vi "Periodic Tasks.vi"(8 "error in":errorcluster) -> ()   [LabVIEW 2015]
doc: "This VI runs in parallel to other tasks. It can contain as many user-defined periodic loops as you need. These can carry out PID or other sorts of timed response."
uses:
  <vilib>/Rock Robotics/WPI/Solenoid/WPI_SolenoidValue.ctl
  Robot Global Data.vi
  <vilib>/Rock Robotics/Network Tables/NT Write Boolean.vi
  <vilib>/Rock Robotics/Network Tables/NT Write Number.vi
  <vilib>/Rock Robotics/WPI/Solenoid/WPI_SolenoidSetEnum.vi
  <vilib>/Rock Robotics/Network Tables/NT Write Raw.vi
  <vilib>/Rock Robotics/Network Tables/NT Write Numeric Array.vi
  <vilib>/Rock Robotics/Network Tables/NT Read Boolean.vi
  <vilib>/Rock Robotics/WPI/Utilities/WPI_GetSetVariantRefNum.vi
panel:
  in  "Trim Speed":dbl
  in  "Rate":dbl min=0.0 max=0.1 step=0.001
  out "Ramp Up":dbl(knob) scale=0.0..1.0
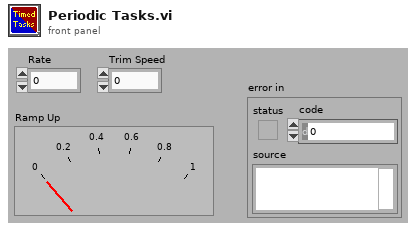
[diagram p1: front panel]
types:
  T1 = typedef "WPI_SolenoidValue.ctl" = enum16{"Off", "On", "Forward", "Reverse"}
  T2 = typedef "WPI_SolenoidDevRef.ctl" = cluster{"DevStatus":errorcluster, "Pneumatics Control Module":u8, "Forward Solenoid Channel":T3, "Reverse Solenoid Channel":T3}
  T3 = typedef "WPI_SolenoidChannel.ctl" = enum8{"Solenoid 0", "Solenoid 1", "Solenoid 2", "Solenoid 3", "Solenoid 4", "Solenoid 5", "Solenoid 6", "Solenoid 7", "Invalid"}
  T4 = typedef "WPI_DigitalInputDevRef.ctl" = cluster{"DevStatus":errorcluster, "DIO Channel":T5}
  T5 = typedef "FPGA_DIOChannel.ctl" = enum8{"DIO 0", "DIO 1", "DIO 2", "DIO 3", "DIO 4", "DIO 5", "DIO 6", "DIO 7", "DIO 8", "DIO 9", "DIO MXP 0", "DIO MXP 1", "DIO MXP 2", "DIO MXP 3", "DIO MXP 4", "DIO MXP 5", "DIO MXP 6", "DIO MXP 7", "DIO MXP 8", "DIO MXP 9", "DIO MXP 10", "DIO MXP 11", "DIO MXP 12", "DIO MXP 13", "DIO MXP 14", "DIO MXP 15", "Invalid"}
  T6 = typedef "WPI_MotorControlDeviceRef.ctl" = cluster{"DeviceStatus":errorcluster, "Type":T7, "PWM":cluster{"PWM Channel":T8, "DeadBand":T9}, "CAN":cluster{"Device Number":u8, "Control Mode":T10, "Semaphore":T11, "Max Vout":dbl, "TalonSRX Control Mode":T12}, "Invert":bool}
  T7 = typedef "WPI_MotorControlType.ctl" = enum16{"PWM", "CAN", "CANTalonSRX"}
  T8 = typedef "FPGA_DIOPWMChannel.ctl" = enum8{"PWM 0", "PWM 1", "PWM 2", "PWM 3", "PWM 4", "PWM 5", "PWM 6", "PWM 7", "PWM 8", "PWM 9", "PWM MXP 0", "PWM MXP 1", "PWM MXP 2", "PWM MXP 3", "PWM MXP 4", "PWM MXP 5", "PWM MXP 6", "PWM MXP 7", "PWM MXP 8", "PWM MXP 9", "Invalid"}
  T9 = typedef "WPI_PWMDeadband.ctl" = cluster{"Name":string, "maxPositivePwm":i32, "minPositivePwm":i32, "centerPwm":i32, "maxNegativePwm":i32, "minNegativePwm":i32, "angularRange":u16}
  T10 = typedef "WPI_CANJaguar_ControlMode.ctl" = enum8{"Percent VBus", "Current", "Speed", "Position", "Voltage"}
  T11 = typedef "Semaphore RefNum" = refnum<k1>
  T12 = typedef "WPI_CANTalonSRX_APIControlMode.ctl" = enum8{"Percent VBus", "Speed", "Position", "Slave", "Unchanged / Invalid", "Voltage Compensation", "Current", "Motion Profile"}
  T13 = typedef "WPI_RobotDriveDevRef.ctl" = cluster{"DevStatus":errorcluster, "Motors[]":T6[], "Square Inputs":bool, "Max Output":dbl}
  T14 = typedef "WPI_DriverStationRobotMode2.ctl" = enum16{"Autonomous Disabled", "Autonomous Enabled", "Teleop Disabled", "Teleop Enabled", "Disconnected", "Finish", "Test Disabled", "Test Enabled", "Emergency Stopped"}
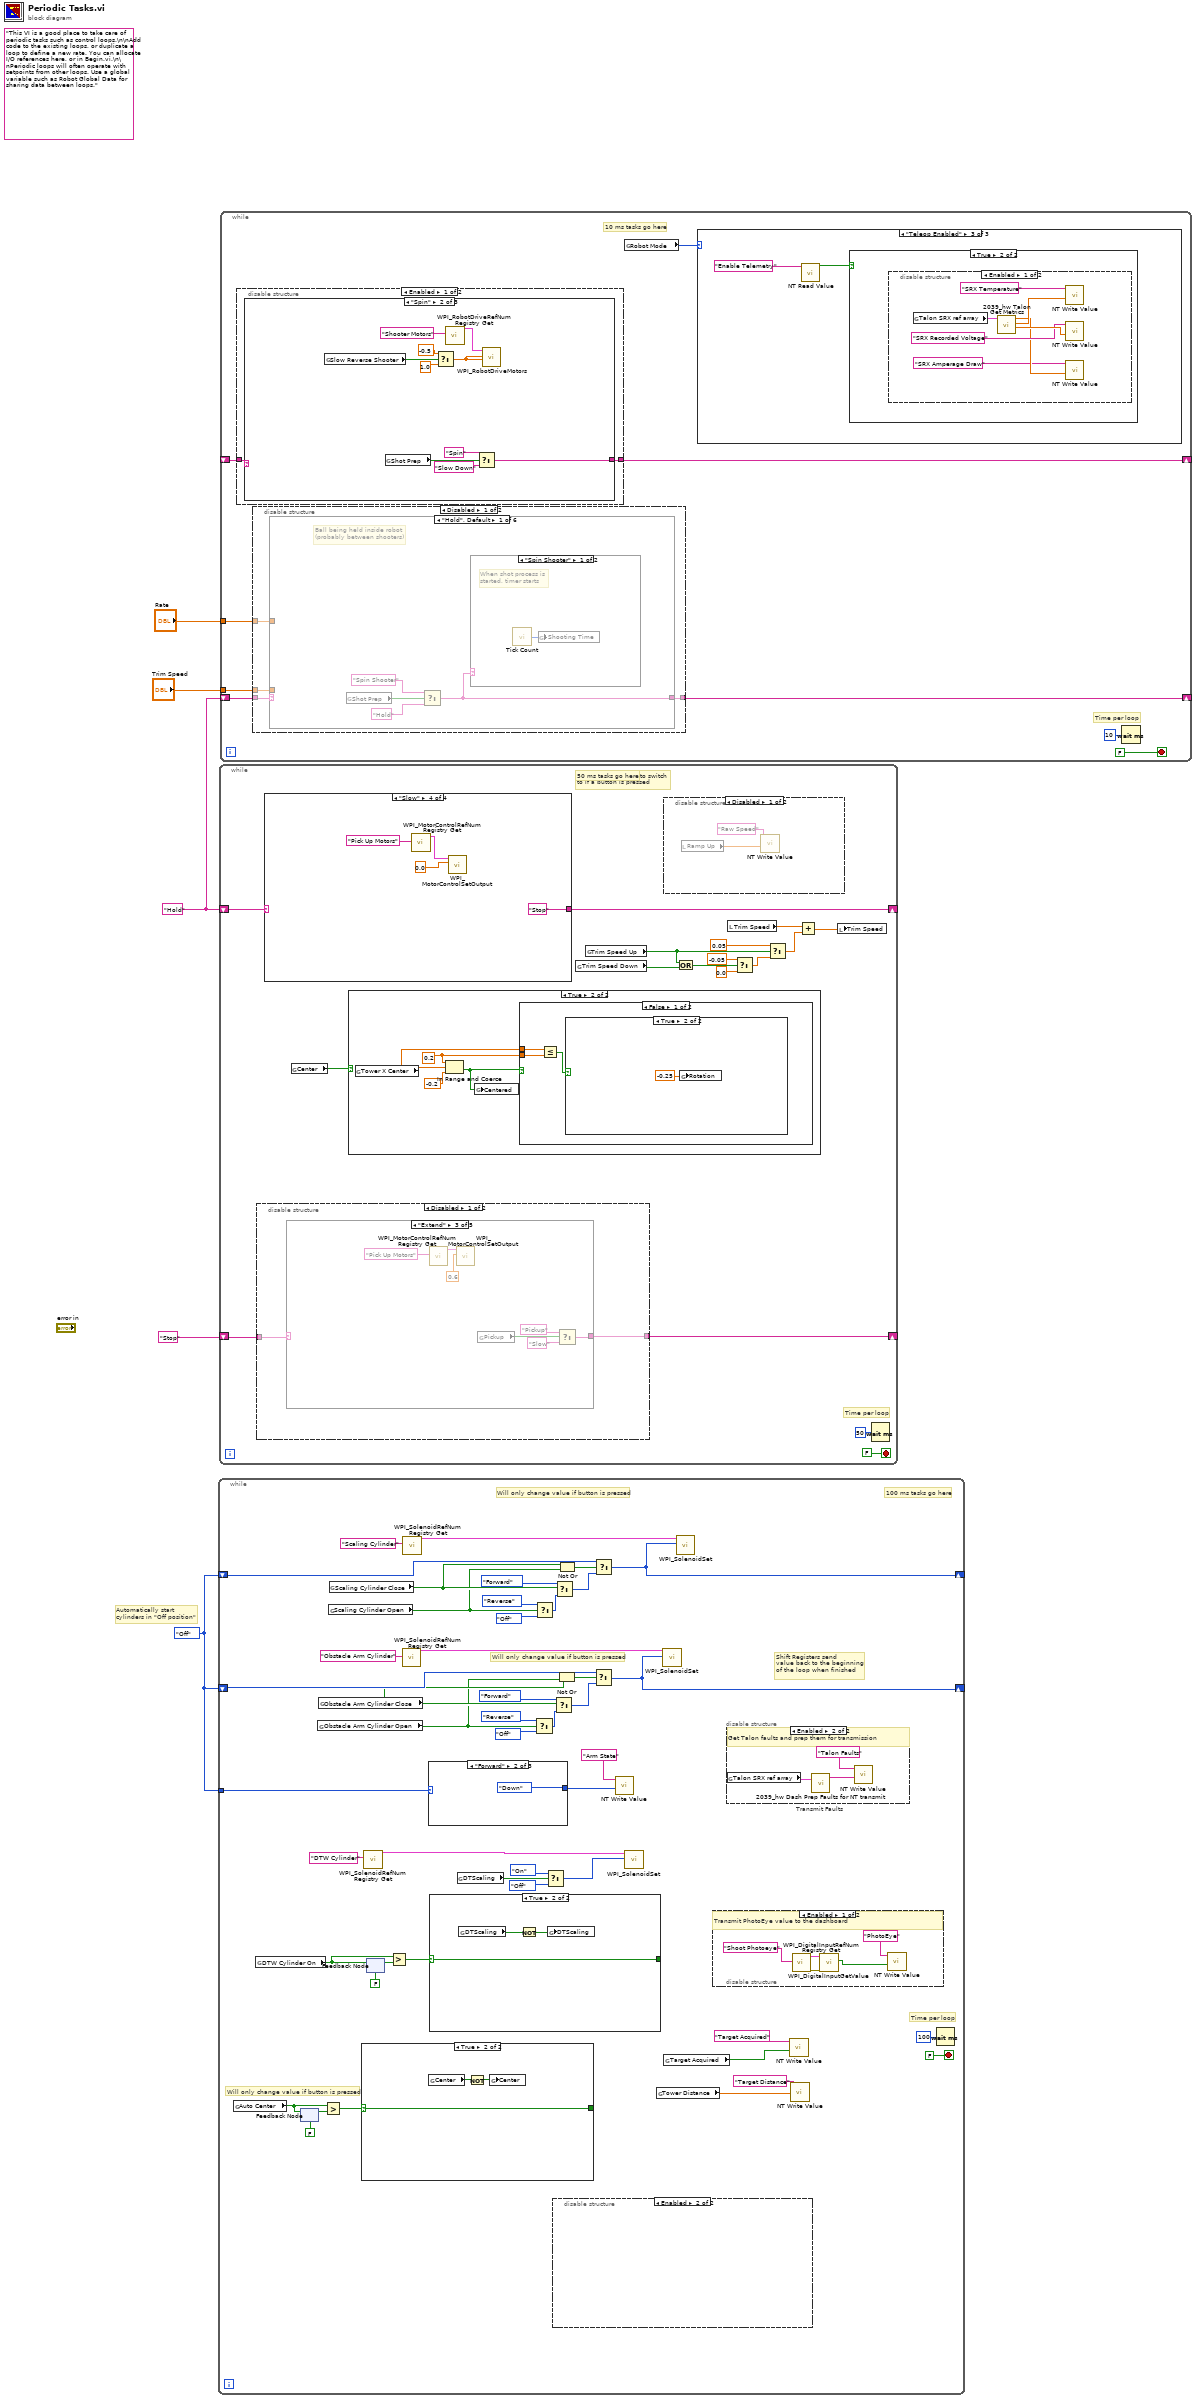
[diagram p0: block diagram]
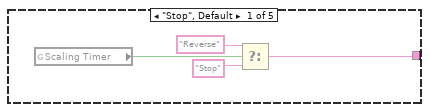
[diagram p2: hidden frame]
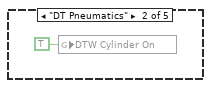
[diagram p3: hidden frame]
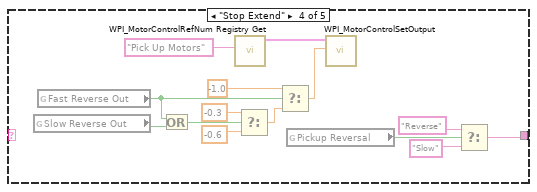
[diagram p4: hidden frame]
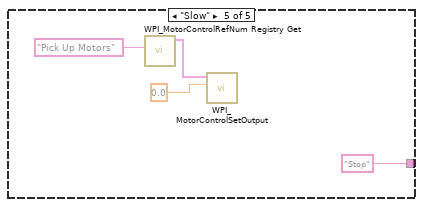
[diagram p5: hidden frame]
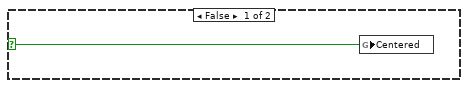
[diagram p8: hidden frame]
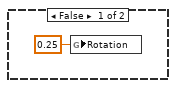
[diagram p9: hidden frame]
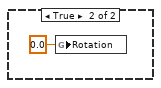
[diagram p10: hidden frame]
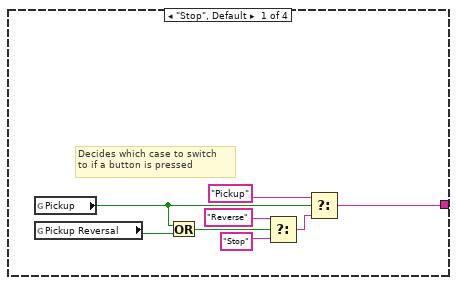
[diagram p11: hidden frame]
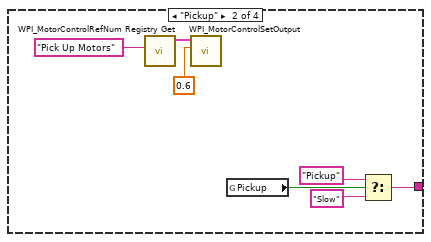
[diagram p12: hidden frame]
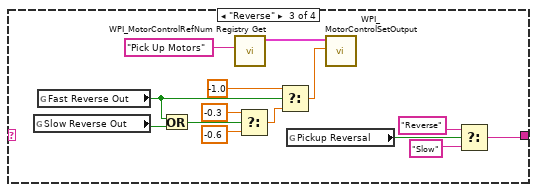
[diagram p13: hidden frame]
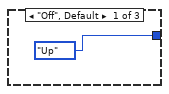
[diagram p18: hidden frame]
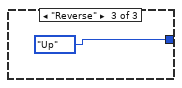
[diagram p19: hidden frame]
diagram:
  w2 = WPI_SolenoidValue."Off" ("Value")
  w4 = "Hold"
  (unwired) "This VI is a good place to take care of periodic tasks such as control loops.\n\nAdd code to the existing loops, or duplicate a loop to define a new rate. You can allocate I/O references here, or in Begin.vi.\n\nPeriodic loops will often operate with setpoints from other loops. Use a global variable such as Robot Global Data for sharing data between loops."
  # "Automatically start \ncylinders in \"Off position\""
  n1 = while {
    shift-right: [w50] -> _
    shift-left: w2 -> [w49]
    shift-right: [w44] -> _
    shift-left: w2 -> [w43]
    tunnel: w2 -> [w23]
    stop <- FALSE stop-if-true
    # "Will only change value if button is pressed"
    # "Will only change value if button is pressed"
    # "Will only change value if button is pressed"
    # "Shift Registers send\nvalue back to the beginning\nof the loop when finished"
    # "Time per loop"
    # "100 ms tasks go here"
    n2 = global read "Robot Global Data.vi" "Auto Center"() -> (w18:bool)
    n3 = global read "Robot Global Data.vi" "DTW Cylinder On"() -> (w9:bool)
    n4 = feedback-in #1(w18) -> ()
    n5 = feedback #1(FALSE ("Auto Center")) -> (w19:bool)
    n6 = global read "Robot Global Data.vi" "Obstacle Arm Cylinder Open"() -> (w33:bool)
    n7 = global read "Robot Global Data.vi" "Obstacle Arm Cylinder Close"() -> (w34:bool)
    n8 = Greater?(x=w18, y=w19) -> (0:w20:bool)
    n9 = global read "Robot Global Data.vi" "Scaling Cylinder Open"() -> (w12:bool)
    n10 = global read "Robot Global Data.vi" "Scaling Cylinder Close"() -> (w24:bool)
    n11 = case shown="True" w20 {
      selector: w20 -> [w68 w71]
      tunnel: [w68 w71] -> _
      frame False {
      }
      frame True {
        n12 = global read "Robot Global Data.vi" "Center"() -> (w69:bool)
        n13 = Not(x=w69) -> (.not. x?=w70:bool)
        n14 = global write "Robot Global Data.vi" "Center"(w70) -> ()
      }
    }
    n15 = call <vilib>:"WPI_SolenoidRefNum Registry Get.vi"("refnum name"="DTW Cylinder") -> ("SolenoidDevRef"=w47:T2)  [unwired: 9 in, 1 out]
    n16 = feedback #2(FALSE ("Auto Center")) -> (w11:bool)
    n17 = feedback-in #2(w9) -> ()
    n18 = Greater?(x=w9, y=w11) -> (0:w6:bool)
    n19 = call <vilib>:"WPI_SolenoidRefNum Registry Get.vi"("refnum name"="Obstacle Arm Cylinder") -> ("SolenoidDevRef"=w37:T2)  [unwired: 9 in, 1 out]
    n20 = call <vilib>:"WPI_SolenoidRefNum Registry Get.vi"("refnum name"="Scaling Cylinder") -> ("SolenoidDevRef"=w27:T2)  [unwired: 9 in, 1 out]
    n21 = case shown="\"Forward\"" w23 {
      tunnel: [enum16{"Up", "Down"}."Up" enum16{"Up", "Down"}."Down" enum16{"Up", "Down"}."Up"] -> w22
      frame "Off", Default {
      }
      frame "Forward" {
      }
      frame "Reverse" {
      }
    }
    n22 = case shown="True" w6 {
      selector: w6 -> [w53 w56]
      tunnel: [w53 w56] -> _
      frame False {
      }
      frame True {
        n23 = global read "Robot Global Data.vi" "DTScaling"() -> (w54:bool)
        n24 = Not(x=w54) -> (.not. x?=w55:bool)
        n25 = global write "Robot Global Data.vi" "DTScaling"(w55) -> ()
      }
    }
    n26 = global read "Robot Global Data.vi" "DTScaling"() -> (w7:bool)
    n27 = Select(t=WPI_SolenoidValue."Reverse" ("Value"), s=w33, f=WPI_SolenoidValue."Off" ("Value")) -> (s? t:f=w39:T1)
    n28 = Select(t=WPI_SolenoidValue."Reverse" ("Value"), s=w12, f=WPI_SolenoidValue."Off" ("Value")) -> (s? t:f=w29:T1)
    n29 = Select(t=WPI_SolenoidValue."On" ("Value"), s=w7, f=WPI_SolenoidValue."Off" ("Value")) -> (s? t:f=w8:T1)
    n30 = disable-structure shown="Enabled" {
      frame Disabled {
      }
      frame Enabled {
      }
    }
    n31 = Select(t=WPI_SolenoidValue."Forward" ("Value"), s=w34, f=w39) -> (s? t:f=w36:T1)
    n32 = Select(t=WPI_SolenoidValue."Forward" ("Value"), s=w24, f=w29) -> (s? t:f=w26:T1)
    n33 = Not Or(1:w33, 2:w34) -> (0:w35:bool)
    n34 = Not Or(1:w12, 2:w24) -> (0:w25:bool)
    n35 = Select(t=w43, s=w35, f=w36) -> (s? t:f=w44:T1)
    n36 = Select(t=w49, s=w25, f=w26) -> (s? t:f=w50:T1)
    n37 = call-poly <vilib>:"NT Write Value.vi"("Numeric"=w22, "Name"="Arm State") -> ()  [unwired: 9 in, 1 out]
    n38 = call-poly <vilib>:"WPI_SolenoidSet.vi"("Value"=w8, "SolenoidDevRef"=w47) -> ()  [unwired: 1 in, 9 out]
    n39 = global read "Robot Global Data.vi" "Tower Distance"() -> (w14:dbl)
    n40 = call-poly <vilib>:"WPI_SolenoidSet.vi"("Value"=w44, "SolenoidDevRef"=w37) -> ()  [unwired: 1 in, 9 out]
    n41 = global read "Robot Global Data.vi" "Target Acquired"() -> (w16:bool)
    n42 = call-poly <vilib>:"WPI_SolenoidSet.vi"("Value"=w50, "SolenoidDevRef"=w27) -> ()  [unwired: 1 in, 9 out]
    n43 = disable-structure shown="Enabled" {
      frame Enabled {
        # "Transmit PhotoEye value to the dashboard"
        n44 = call <vilib>:"WPI_DigitalInputRefNum Registry Get.vi"("refnum name"="Shoot Photoeye") -> ("error out"=w59:errorcluster, "DigitalInputDevRef"=w60:T4)  [unwired: 9 in]
        n45 = call <vilib>:"WPI_DigitalInputGetValue.vi"("error in (no error)"=w59, "DigitalInputDevRef"=w60) -> ("Value"=w58:bool)  [unwired: 7 in, 2 out]
        n46 = call-poly <vilib>:"NT Write Value.vi"("Boolean"=w58, "Name"="PhotoEye") -> ()  [unwired: 9 in, 1 out]
      }
      frame Disabled {
      }
    }
    n47 = disable-structure "Transmit Faults" shown="Enabled" {
      frame Disabled {
      }
      frame Enabled {
        # "Get Talon faults and prep them for transmission"
        n48 = global read "Robot Global Data.vi" "Talon SRX ref array"() -> (w64:T6[])
        n49 = call "2039_hw Dash Prep Faults for NT transmit.vi"("Talon SRX ref array"=w64) -> ("data string"=w62:string)  [unwired: 1 in, 1 out]
        n50 = call-poly <vilib>:"NT Write Value.vi"("Raw"=w62, "Name"="Talon Faults") -> ()  [unwired: 9 in, 1 out]
      }
    }
    n51 = call-poly <vilib>:"NT Write Value.vi"("Boolean"=w16, "Name"="Target Acquired") -> ()  [unwired: 9 in, 1 out]
    n52 = call-poly <vilib>:"NT Write Value.vi"("Numeric"=w14, "Name"="Target Distance") -> ()  [unwired: 9 in, 1 out]
    n53 = Wait (ms)(milliseconds to wait=u32 100) -> ()  [unwired: 1 out]
  }
  n54 = while {
    shift-right: [w85] -> _
    shift-left: w4 -> [w86]
    shift-right: [w72] -> _
    shift-left: "Stop" -> [w73]
    stop <- FALSE stop-if-true
    # "Decides which case to switch \nto if a button is pressed"
    # "Time per loop"
    # "50 ms tasks go here"
    n55 = disable-structure shown="Disabled" {
      disable-tunnel: w73 -> [w90 _]
      disable-tunnel: [w89 _] -> w72
      frame Disabled {
        n56 = case shown="\"Extend\"" w90 {
          tunnel: [w92 _ w99 w112 "Stop" ("f")] -> w89
          frame "Stop", Default {
            n57 = global read "Robot Global Data.vi" "Scaling Timer"() -> (w91:bool)
            n58 = Select(t="Reverse", s=w91, f="Stop") -> (s? t:f=w92:string)
          }
          frame "DT Pneumatics" {
            n59 = global write "Robot Global Data.vi" "DTW Cylinder On"(TRUE ("DTW Cylinder On")) -> ()
          }
          frame "Extend" {
            n60 = call <vilib>:"WPI_MotorControlRefNum Registry Get.vi"("refnum name"="Pick Up Motors") -> ("MotorControlDevRef"=w96:T6)  [unwired: 9 in, 1 out]
            n61 = call <vilib>:"WPI_MotorControlSetOutput.vi"("Output"=0.6 ("RightSpeed"), "MotorControlDevRef"=w96) -> ()  [unwired: 7 in, 3 out]
            n62 = global read "Robot Global Data.vi" "Pickup"() -> (w101:bool)
            n63 = Select(t="Pickup", s=w101, f="Slow") -> (s? t:f=w99:string)
          }
          frame "Stop Extend" {
            n64 = global read "Robot Global Data.vi" "Slow Reverse Out"() -> (w109:bool)
            n65 = global read "Robot Global Data.vi" "Fast Reverse Out"() -> (w107:bool)
            n66 = Or(x=w107, y=w109) -> (x .or. y?=w108:bool)
            n67 = call <vilib>:"WPI_MotorControlRefNum Registry Get.vi"("refnum name"="Pick Up Motors") -> ("MotorControlDevRef"=w111:T6)  [unwired: 9 in, 1 out]
            n68 = Select(t=-0.3, s=w108, f=-0.6) -> (s? t:f=w110:dbl)
            n69 = Select(t=-1.0, s=w107, f=w110) -> (s? t:f=w103:dbl)
            n70 = global read "Robot Global Data.vi" "Pickup Reversal"() -> (w114:bool)
            n71 = call <vilib>:"WPI_MotorControlSetOutput.vi"("Output"=w103, "MotorControlDevRef"=w111) -> ()  [unwired: 7 in, 3 out]
            n72 = Select(t="Reverse", s=w114, f="Slow") -> (s? t:f=w112:string)
          }
          frame "Slow" {
            n73 = call <vilib>:"WPI_MotorControlRefNum Registry Get.vi"("refnum name"="Pick Up Motors") -> ("MotorControlDevRef"=w117:T6)  [unwired: 9 in, 1 out]
            n74 = call <vilib>:"WPI_MotorControlSetOutput.vi"("Output"=0.0 ("RightSpeed"), "MotorControlDevRef"=w117) -> ()  [unwired: 7 in, 3 out]
          }
        }
      }
      frame Enabled {
      }
    }
    n75 = case shown="\"Slow\"" w86 {
      tunnel: [w134 w145 w158 "Stop" ("f")] -> w85
      frame "Stop", Default {
        # "Decides which case to switch \nto if a button is pressed"
        n76 = global read "Robot Global Data.vi" "Pickup"() -> (w136:bool)
        n77 = global read "Robot Global Data.vi" "Pickup Reversal"() -> (w135:bool)
        n78 = Or(x=w136, y=w135) -> (x .or. y?=w137:bool)
        n79 = Select(t="Reverse", s=w137, f="Stop") -> (s? t:f=w141:string)
        n80 = Select(t="Pickup", s=w136, f=w141) -> (s? t:f=w134:string)
      }
      frame "Pickup" {
        n81 = call <vilib>:"WPI_MotorControlRefNum Registry Get.vi"("refnum name"="Pick Up Motors") -> ("MotorControlDevRef"=w142:T6)  [unwired: 9 in, 1 out]
        n82 = call <vilib>:"WPI_MotorControlSetOutput.vi"("Output"=0.6 ("RightSpeed"), "MotorControlDevRef"=w142) -> ()  [unwired: 7 in, 3 out]
        n83 = global read "Robot Global Data.vi" "Pickup"() -> (w147:bool)
        n84 = Select(t="Pickup", s=w147, f="Slow") -> (s? t:f=w145:string)
      }
      frame "Reverse" {
        n85 = global read "Robot Global Data.vi" "Slow Reverse Out"() -> (w155:bool)
        n86 = global read "Robot Global Data.vi" "Fast Reverse Out"() -> (w153:bool)
        n87 = Or(x=w153, y=w155) -> (x .or. y?=w154:bool)
        n88 = call <vilib>:"WPI_MotorControlRefNum Registry Get.vi"("refnum name"="Pick Up Motors") -> ("MotorControlDevRef"=w157:T6)  [unwired: 9 in, 1 out]
        n89 = Select(t=-0.3, s=w154, f=-0.6) -> (s? t:f=w156:dbl)
        n90 = Select(t=-1.0, s=w153, f=w156) -> (s? t:f=w149:dbl)
        n91 = global read "Robot Global Data.vi" "Pickup Reversal"() -> (w160:bool)
        n92 = call <vilib>:"WPI_MotorControlSetOutput.vi"("Output"=w149, "MotorControlDevRef"=w157) -> ()  [unwired: 7 in, 3 out]
        n93 = Select(t="Reverse", s=w160, f="Slow") -> (s? t:f=w158:string)
      }
      frame "Slow" {
        n94 = call <vilib>:"WPI_MotorControlRefNum Registry Get.vi"("refnum name"="Pick Up Motors") -> ("MotorControlDevRef"=w163:T6)  [unwired: 9 in, 1 out]
        n95 = call <vilib>:"WPI_MotorControlSetOutput.vi"("Output"=0.0 ("RightSpeed"), "MotorControlDevRef"=w163) -> ()  [unwired: 7 in, 3 out]
      }
    }
    n96 = global read "Robot Global Data.vi" "Center"() -> (w74:bool)
    n97 = case shown="True" w74 {
      selector: w74 -> [w123 _]
      frame False {
        n98 = global write "Robot Global Data.vi" "Centered"(w123) -> ()
      }
      frame True {
        w125 = 0.2 ("y")
        n99 = global read "Robot Global Data.vi" "Tower X Center"() -> (w126:dbl)
        n100 = In Range and Coerce(upper limit=w125, x=w126, lower limit=-0.2 ("y")) -> (In Range?=w124:bool)  [unwired: 1 out]
        n101 = global write "Robot Global Data.vi" "Centered"(w124) -> ()
        n102 = case shown="False" w124 {
          tunnel: w126 -> [w129 _]
          tunnel: w125 -> [w128 _]
          frame False {
            n103 = Less Or Equal?(x=w129, y=w128) -> (x <= y?=w130:bool)
            n104 = case shown="True" w130 {
              frame False {
                n105 = global write "Robot Global Data.vi" "Rotation"(0.25 ("Rotation")) -> ()
              }
              frame True {
                n106 = global write "Robot Global Data.vi" "Rotation"(-0.25 ("Rotation")) -> ()
              }
            }
          }
          frame True {
            n107 = global write "Robot Global Data.vi" "Rotation"(0.0 ("Rotation")) -> ()
          }
        }
      }
    }
    n108 = global read "Robot Global Data.vi" "Trim Speed Down"() -> (w83:bool)
    n109 = global read "Robot Global Data.vi" "Trim Speed Up"() -> (w81:bool)
    n110 = disable-structure shown="Disabled" {
      frame Disabled {
        n111 = local read "Ramp Up"() -> (w121:dbl)
        n112 = call-poly <vilib>:"NT Write Value.vi"("Numeric"=w121, "Name"="Raw Speed") -> ()  [unwired: 9 in, 1 out]
      }
      frame Enabled {
      }
    }
    n113 = Or(x=w81, y=w83) -> (x .or. y?=w82:bool)
    n114 = local read "Trim Speed"() -> (w76:dbl)
    n115 = Select(t=-0.05, s=w82, f=0.0) -> (s? t:f=w84:dbl)
    n116 = Select(t=0.05, s=w81, f=w84) -> (s? t:f=w77:dbl)
    n117 = Add(x=w76, y=w77) -> (x+y=w75:dbl)
    n118 = local write "Trim Speed"(w75) -> ()
    n119 = Wait (ms)(milliseconds to wait=u32 50) -> ()  [unwired: 1 out]
  }
  n120 = while {
    shift-right: [w173] -> _
    shift-left: _ -> [w169]
    tunnel: "Rate" -> [w172]
    shift-right: [w171] -> _
    shift-left: w4 -> [w170]
    tunnel: "Trim Speed" -> [w168]
    stop <- FALSE stop-if-true
    # "10 ms tasks go here"
    # "Time per loop"
    n121 = disable-structure shown="Enabled" {
      disable-tunnel: [w194 _] -> w173
      disable-tunnel: w169 -> [w193 _]
      frame Enabled {
        n122 = case shown="\"Spin\"" w193 {
          tunnel: [w195 w207 w210] -> w194
          frame "Hold", Default {
            n123 = global read "Robot Global Data.vi" "Shot Prep"() -> (w198:bool)
            n124 = Select(t="Spin", s=w198, f="Hold") -> (s? t:f=w195:string)
            n125 = case shown="\"Spin\"" w195 {
              frame "Spin" {
                n126 = call "Tick Count10"() -> ("Tick Count(mSec)"=w199:u32)
                n127 = global write "Robot Global Data.vi" "Shooting Time"(w199) -> ()
              }
              frame "Hold", Default {
              }
            }
          }
          frame "Spin" {
            n128 = global read "Robot Global Data.vi" "Slow Reverse Shooter"() -> (w201:bool)
            n129 = global read "Robot Global Data.vi" "Shot Prep"() -> (w206:bool)
            n130 = Select(t=-0.5, s=w201, f=1.0 ("RightSpeed")) -> (s? t:f=w200:dbl)
            n131 = call <vilib>:"WPI_RobotDriveRefNum Registry Get.vi"("refnum name"="Shooter Motors") -> ("RobotDriveDevRef"=w204:T13)  [unwired: 9 in, 1 out]
            n132 = Select(t="Spin", s=w206, f="Slow Down") -> (s? t:f=w207:string)
            n133 = call <vilib>:"WPI_RobotDriveMotors.vi"("RightSpeed"=w200, "LeftSpeed"=w200, "RobotDriveDevRef"=w204) -> ()  [unwired: 6 in, 3 out]
          }
          frame "Slow Down" {
            w218 = 0.0 ("RightSpeed")
            n134 = global read "Robot Global Data.vi" "Shooting Time"() -> (w211:i32)
            n135 = call "Tick Count14"() -> ("Tick Count(mSec)"=w212:u32)
            n136 = Subtract(x=w212, y=w211) -> (x-y=w215:u32)
            n137 = call <vilib>:"WPI_RobotDriveRefNum Registry Get.vi"("refnum name"="Shooter Motors") -> ("RobotDriveDevRef"=w219:T13)  [unwired: 9 in, 1 out]
            n138 = call <vilib>:"WPI_RobotDriveMotors.vi"("RightSpeed"=w218, "LeftSpeed"=w218, "RobotDriveDevRef"=w219) -> ()  [unwired: 6 in, 3 out]
            n139 = Greater?(x=w215, y=u32 10) -> (0:w216:bool)
            n140 = Select(t="Hold", s=w216, f="Slow Down") -> (s? t:f=w210:string)
          }
        }
      }
      frame Disabled {
      }
    }
    n141 = disable-structure shown="Disabled" {
      disable-tunnel: w172 -> [w224 _]
      disable-tunnel: [w223 _] -> w171
      disable-tunnel: w170 -> [w222 _]
      disable-tunnel: w168 -> [w221 _]
      frame Disabled {
        n142 = case shown="\"Hold\", Default" w222 {
          tunnel: [w225 w233 w253 w263 w270 "Hold" ("t")] -> w223
          tunnel: w224 -> [_ _ w249 _ _ _]
          tunnel: w221 -> [_ _ w243 _ _ _]
          frame "Hold", Default {
            # "Ball being held inside robot \n(probably between shooters)"
            n143 = global read "Robot Global Data.vi" "Shot Prep"() -> (w228:bool)
            n144 = Select(t="Spin Shooter", s=w228, f="Hold") -> (s? t:f=w225:string)
            n145 = case shown="\"Spin Shooter\"" w225 {
              frame "Spin Shooter" {
                # "When shot process is \nstarted, timer starts"
                n146 = call "Tick Count"() -> ("Tick Count(mSec)"=w229:u32)
                n147 = global write "Robot Global Data.vi" "Shooting Time"(w229) -> ()
              }
              frame "Hold", Default {
                # "Do Nothing"
              }
            }
          }
          frame "Unload Ball" {
            w230 = -0.1 ("RightSpeed")
            # "Move ball out of \nshooters before spinup"
            n148 = global read "Robot Global Data.vi" "Shooting Time"() -> (w234:i32)
            n149 = call <vilib>:"WPI_RobotDriveRefNum Registry Get.vi"("refnum name"="Shooter Motors") -> ("RobotDriveDevRef"=w231:T13)  [unwired: 9 in, 1 out]
            n150 = call "Tick Count2"() -> ("Tick Count(mSec)"=w235:u32)
            n151 = Subtract(x=w235, y=w234) -> (x-y=w238:u32)
            n152 = call <vilib>:"WPI_RobotDriveMotors.vi"("RightSpeed"=w230, "LeftSpeed"=w230, "RobotDriveDevRef"=w231) -> ()  [unwired: 6 in, 3 out]
            n153 = Greater?(x=w238, y=u32 250) -> (0:w239:bool)
            n154 = Select(t="Spin Shooter", s=w239, f="Unload Ball") -> (s? t:f=w233:string)
          }
          frame "Spin Shooter" {
            # "Ramp up shooters\nto desired speed"
            # "Will switch case when at desired speed"
            # "Continues to ramp up if NOT \ngreater than/equal to rate needed"
            n155 = global read "Robot Global Data.vi" "High Shot Speed"() -> (w247:bool)
            n156 = local read "Ramp Up"() -> (w252:dbl)
            n157 = Add(x=0.75 ("y"), y=w243) -> (x+y=w245:dbl)
            n158 = Add(x=w243, y=0.45) -> (x+y=w244:dbl)
            n159 = Select(t=w245, s=w247, f=w244) -> (s? t:f=w248:dbl)
            n160 = Greater Or Equal?(x=w252, y=w248) -> (x >= y?=w250:bool)
            n161 = Not(x=w250) -> (.not. x?=w251:bool)
            n162 = case shown="True" w251 {
              tunnel: w249 -> [_ w261]
              tunnel: w252 -> [_ w260]
              frame False {
                # "If at correct speed, stay at that speed"
                n163 = local read "Ramp Up"() -> (w258:dbl)
                n164 = local write "Ramp Up"(w258) -> ()
              }
              frame True {
                # "Adds rate to current \nramping speed"
                n165 = Add(x=w260, y=w261) -> (x+y=w259:dbl)
                n166 = local write "Ramp Up"(w259) -> ()
              }
            }
            n167 = local read "Ramp Up"() -> (w246:dbl)
            "Ramp Up" <- w246
            n168 = call <vilib>:"WPI_RobotDriveRefNum Registry Get.vi"("refnum name"="Shooter Motors") -> ("RobotDriveDevRef"=w254:T13)  [unwired: 9 in, 1 out]
            n169 = call <vilib>:"WPI_RobotDriveMotors.vi"("RightSpeed"=w246, "LeftSpeed"=w246, "RobotDriveDevRef"=w254) -> ()  [unwired: 6 in, 3 out]
            n170 = Select(t="Shot Prep", s=w250, f="Spin Shooter") -> (s? t:f=w253:string)
          }
          frame "Shot Prep" {
            # "Added to allow you to stop the \nspinup process midway if needed"
            n171 = global read "Robot Global Data.vi" "Shot Prep"() -> (w264:bool)
            n172 = global read "Robot Global Data.vi" "Pickup"() -> (w262:bool)
            n173 = Or(x=w262, y=w264) -> (x .or. y?=w265:bool)
            n174 = Select(t="Slow Down", s=w265, f="Shot Prep") -> (s? t:f=w269:string)
            n175 = Select(t="Take Shot", s=w262, f=w269) -> (s? t:f=w263:string)
          }
          frame "Take Shot" {
            w279 = 0.6 ("RightSpeed")
            # "Slow down after 750ms"
            # "Throws the ball through\nshooter motors"
            n176 = global read "Robot Global Data.vi" "Shooting Time"() -> (w272:i32)
            n177 = call "Tick Count3"() -> ("Tick Count(mSec)"=w273:u32)
            n178 = call <vilib>:"WPI_RobotDriveRefNum Registry Get.vi"("refnum name"="Shooter Motors") -> ("RobotDriveDevRef"=w278:T13)  [unwired: 9 in, 1 out]
            n179 = Subtract(x=w273, y=w272) -> (x-y=w275:u32)
            n180 = call <vilib>:"WPI_RobotDriveMotors.vi"("RightSpeed"=w279, "LeftSpeed"=w279, "RobotDriveDevRef"=w278) -> ()  [unwired: 6 in, 3 out]
            n181 = Greater?(x=w275, y=u32 750) -> (0:w276:bool)
            n182 = Select(t="Slow Down", s=w276, f="Take Shot") -> (s? t:f=w270:string)
          }
          frame "Slow Down" {
            w284 = 0.0 ("RightSpeed")
            # "Slow down the\nmotors to 0"
            n183 = call <vilib>:"WPI_RobotDriveRefNum Registry Get.vi"("refnum name"="Shooter Motors") -> ("RobotDriveDevRef"=w283:T13)  [unwired: 9 in, 1 out]
            n184 = call <vilib>:"WPI_RobotDriveMotors.vi"("RightSpeed"=w284, "LeftSpeed"=w284, "RobotDriveDevRef"=w283) -> ()  [unwired: 6 in, 3 out]
          }
        }
      }
      frame Enabled {
      }
    }
    n185 = global read "Robot Global Data.vi" "Robot Mode"() -> (w167:T14)
    n186 = case shown="\"Teleop Enabled\"" w167 {
      frame "Test Disabled", Default {
        # "If robot is not in test mode, wait 1 ms so the VI does not yield the CPU.  That would be bad."
        n187 = Wait (ms)(milliseconds to wait=u32 1) -> ()  [unwired: 1 out]
      }
      frame "Test Enabled" {
        # "If we're in test mode, or selectively in teleop mode,\nsend Talon telemetry to the dashboard."
        n188 = disable-structure shown="Enabled" {
          frame Enabled {
            n189 = global read "Robot Global Data.vi" "Talon SRX ref array"() -> (w177:T6[])
            n190 = call "2039_hw Talon Get Metrics.vi"("Talon SRX ref array"=w177) -> ("Vbat"=w183:dbl[], "Temperature"=w181:dbl[], "Amperage Draw"=w179:dbl[])  [unwired: 8 in]
            n191 = call-poly <vilib>:"NT Write Value.vi"("Numeric Array"=w181, "Name"="SRX Temperature") -> ()  [unwired: 9 in, 1 out]
            n192 = call-poly <vilib>:"NT Write Value.vi"("Numeric Array"=w183, "Name"="SRX Recorded Voltage") -> ()  [unwired: 9 in, 1 out]
            n193 = call-poly <vilib>:"NT Write Value.vi"("Numeric Array"=w179, "Name"="SRX Amperage Draw") -> ()  [unwired: 9 in, 1 out]
          }
          frame Disabled {
          }
        }
      }
      frame "Teleop Enabled" {
        n194 = call-poly <vilib>:"NT Read Value.vi"("Name"="Enable Telemetry") -> ("Boolean"=w184:bool)  [unwired: 9 in, 1 out]
        n195 = case shown="True" w184 {
          frame False {
          }
          frame True {
            n196 = disable-structure shown="Enabled" {
              frame Enabled {
                n197 = global read "Robot Global Data.vi" "Talon SRX ref array"() -> (w186:T6[])
                n198 = call "2039_hw Talon Get Metrics.vi"("Talon SRX ref array"=w186) -> ("Vbat"=w192:dbl[], "Temperature"=w190:dbl[], "Amperage Draw"=w188:dbl[])  [unwired: 8 in]
                n199 = call-poly <vilib>:"NT Write Value.vi"("Numeric Array"=w190, "Name"="SRX Temperature") -> ()  [unwired: 9 in, 1 out]
                n200 = call-poly <vilib>:"NT Write Value.vi"("Numeric Array"=w192, "Name"="SRX Recorded Voltage") -> ()  [unwired: 9 in, 1 out]
                n201 = call-poly <vilib>:"NT Write Value.vi"("Numeric Array"=w188, "Name"="SRX Amperage Draw") -> ()  [unwired: 9 in, 1 out]
              }
              frame Disabled {
              }
            }
          }
        }
      }
    }
    n202 = Wait (ms)(milliseconds to wait=u32 10) -> ()  [unwired: 1 out]
  }
